vi "数据转移.vi"(6 "原表名":string, 7 "新表名":string, 8 "error in (no error)":errorcluster, 11 "数据库连接引用 i":T1) -> (0 "error out":errorcluster, 3 "数据库连接引用 o":T1, 5 "保留数据？":bool)   [LabVIEW 2017]
uses:
  <vilib>/addons/database/Connection.llb/Conn ObjectReference.ctl
  <vilib>/addons/database/Connection.llb/Conn Execute.vi
  <vilib>/addons/database/NI_Database_API.lvlib
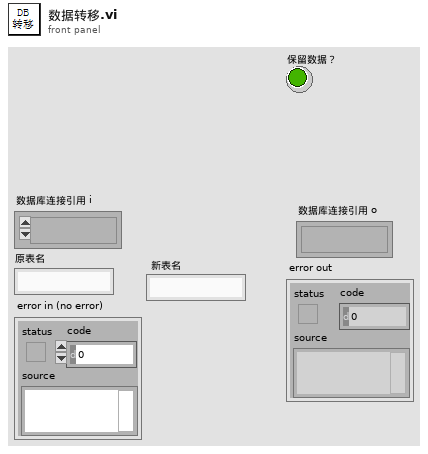
[diagram p1: front panel]
types:
  T1 = typedef "NI_Database_API.lvlib/Conn ObjectReference.ctl" = refnum<k1>
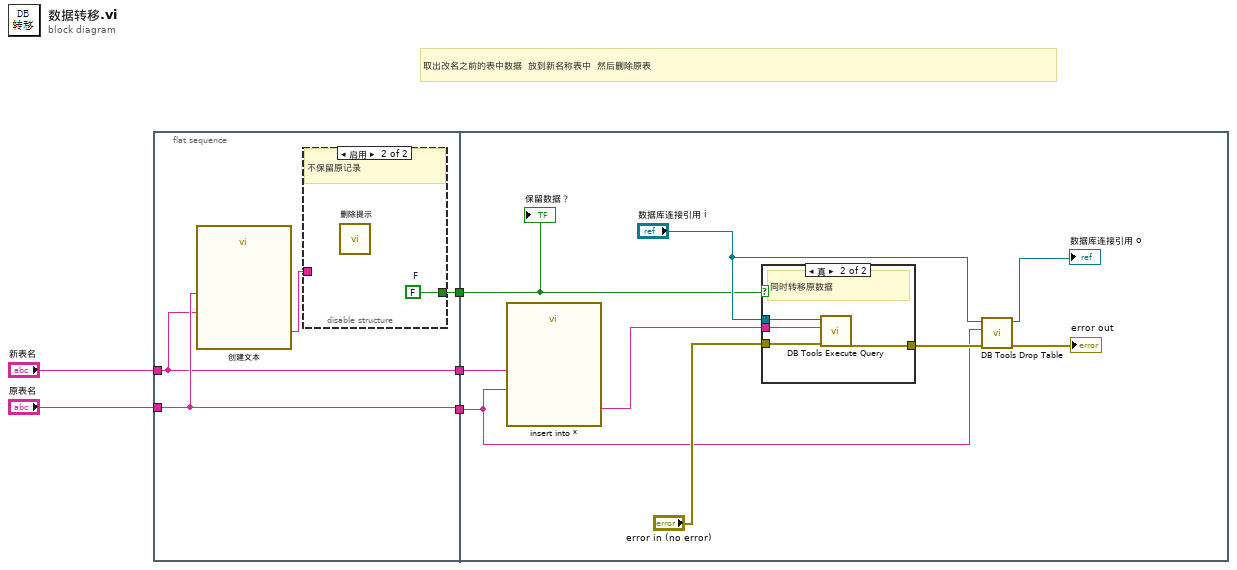
[diagram p0: block diagram]
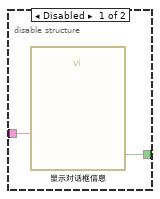
[diagram p2: hidden frame]
diagram:
  # "取出改名之前的表中数据  放到新名称表中  然后删除原表"
  n1 = flat-sequence {
    tunnel: [w8] -> w5
    tunnel: "新表名" -> [w8]
    tunnel: [w9] -> w3
    tunnel: "原表名" -> [w9]
    tunnel: [w6] -> w1
    tunnel: w5 -> [w15]
    tunnel: w3 -> [w14]
    tunnel: w1 -> [w13]
    frame #0 {
      n2 = call "创建文本"("原名称"=w9, "新名称"=w8) -> ("Result"=w7:string)  [unwired: 12 in, 1 out]
      n3 = disable-structure shown="启用" {
        disable-tunnel: w7 -> [w11 _]
        disable-tunnel: [w10 w12] -> w6
        frame Disabled {
          n4 = call "显示对话框信息"("Message"=w11) -> ("确定"=w10:bool)  [unwired: 9 in, 1 out]
        }
        frame Enabled {
          w12 = FALSE  # F
          # "不保留原记录"
          n5 = call "删除提示"() -> ()  [unwired: 10 in, 2 out]
        }
      }
    }
    frame #1 {
      n6 = call "insert into *"("新表名"=w15, "原表名"=w14) -> ("Result"=w21:string)  [unwired: 12 in, 1 out]
      n7 = case shown="真" w13 {
        tunnel: w21 -> [_ w26]
        tunnel: "error in (no error)" -> [w22 w25]
        tunnel: [w22 w24] -> w19
        tunnel: "数据库连接引用 i" -> [_ w23]
        frame False {
        }
        frame True {
          # "同时转移原数据"
          n8 = call-poly <vilib>:"DB Tools Execute Query.vi"("error in (no error)"=w25, "SQL query"=w26, "connection reference"=w23) -> ("error out"=w24:errorcluster)  [unwired: 5 in, 1 out]
        }
      }
      n9 = call <vilib>:"DB Tools Drop Table.vi"("error in (no error)"=w19, "table"=w14, "connection reference"="数据库连接引用 i") -> ("error out"=→"error out":errorcluster, "connection reference out"=→"数据库连接引用 o":T1)  [unwired: 5 in]
      "保留数据？" <- w13
    }
  }
